vi "SetLayout.vi"(7 "PanelVIRef":refnum<vi>, 8 "ErrorIn":errorcluster, 9 "SubPanels":refnum<vi>[](array[refnum]), 10 "Labels":string[](array[string]), 11 "ReferenceIn":refnum<class "MasterGUI.lvclass">) -> (0 "ErrorOut":errorcluster, 3 "ReferenceIn":refnum<class "MasterGUI.lvclass">)   [LabVIEW 2021, in "MasterGUI.lvclass"]
uses:
  MasterGUI.lvclass
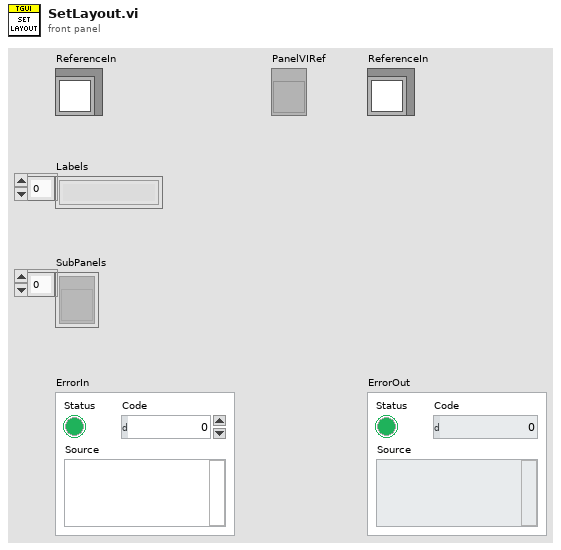
[diagram p1: front panel]
types:
  T1 = typedef "MasterGUI.lvclass/ObjectAttributes.ctl" = cluster{"Interfaces":cluster{"Dummy":refnum<class>}, "Locals":cluster{"MainGUIActive":refnum<queue>, "MainPanel":refnum<vi>, "LayoutPanel":cluster{"PanelVIRef":refnum<vi>, "Labels":string[], "SubPanels":refnum<vi>[]}, "MenuTree":T2[], "Menu":refnum<k9>}, "Persistent":cluster{"StaticDocking":cluster{"ObjectLabel":string, "SubPanelLabel":string}[], "WindowsTitle":string, "AdditionalMenuItems":T2[], "TraceObjectName":string}}
  T2 = typedef "MasterGUI.lvclass/MenuItem.ctl" = cluster{"Parent":string, "Items":string[], "ShortCuts":cluster{"IncludeShiftKey":bool, "IncludeCtrlKey":bool, "ShortcutKey":string}[]}
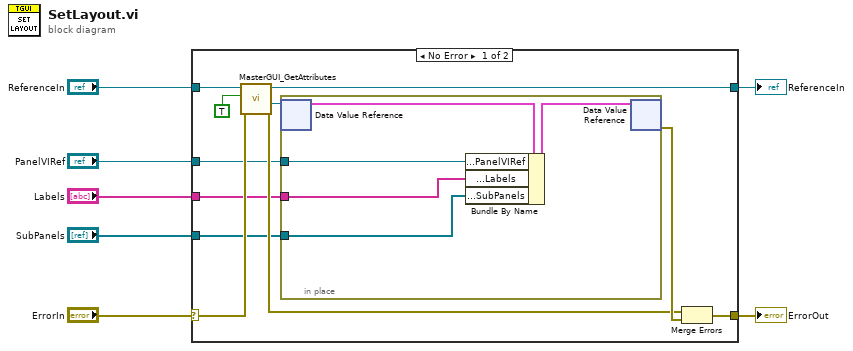
[diagram p0: block diagram]
diagram:
  n1 = case shown="No Error" "ErrorIn" {
    selector: "ErrorIn" -> [w18 w25]
    tunnel: [w15 w25] -> w6
    tunnel: [w13 w24] -> w4
    tunnel: "ReferenceIn" -> [w14 w24]
    tunnel: "SubPanels" -> [w10 _]
    tunnel: "Labels" -> [w9 _]
    tunnel: "PanelVIRef" -> [w8 _]
    frame No Error {
      n2 = call "MasterGUI_GetAttributes.vi"("ErrorIn"=w18, "OnlyGetDvrReference(False)"=TRUE, "ReferenceIn"=w14) -> ("ErrorOut"=w16:errorcluster, "DataRef"=w11:refnum<data-value>, "ReferenceOut"=w13:refnum<class "MasterGUI.lvclass">)  [unwired: 5 in, 1 out]
      n3 = in-place {
        in-place-border: w10 -> [w21]
        in-place-border: w9 -> [w20]
        in-place-border: w8 -> [w19]
        n4 = in-place-dvr #1(w11) -> (w22:T1)  [unwired: 1 out]
        n5 = Bundle By Name(cluster=w22, "Locals.LayoutPanel.PanelVIRef"=w19, "Locals.LayoutPanel.Labels"=w20, "Locals.LayoutPanel.SubPanels"=w21) -> (w23:T1)
        n6 = in-place-dvr #1(w23) -> (w17:errorcluster)  [unwired: 1 out]
      }
      n7 = Merge Errors(w16, w17) -> (w15:errorcluster)
    }
    frame Error {
    }
  }
  "ErrorOut" <- w6
  "ReferenceIn" <- w4
